vi "Await Queue Data Float.vi"(9 "Array":dbl[][](array[numeric]), 10 "Num Elements":i32, 11 "Spare Queue Float":refnum<queue>) -> (3 "Array Out":dbl[][](array[numeric]))   [LabVIEW 2018]
uses:
  Floating Pixel Data STYP.ctl
  Coordinate STYP.ctl
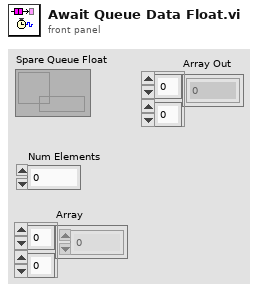
[diagram p1: front panel]
types:
  T1 = typedef "Floating Pixel Data STYP.ctl" = cluster{"Value":dbl, "Coordinate":T2}
  T2 = typedef "Coordinate STYP.ctl" = cluster{"X":i32, "Y":i32}
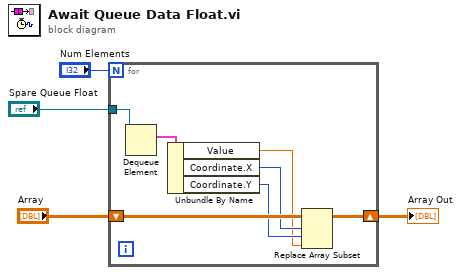
[diagram p0: block diagram]
diagram:
  n1 = for {
    N: "Num Elements" -> [_]
    tunnel: "Spare Queue Float" -> [w11]
    shift-right: [w5] -> w2
    shift-left: "Array" -> [w9]
    n2 = Dequeue Element(queue=w11) -> (element=w10:T1)  [unwired: 2 in, 3 out]
    n3 = Unbundle By Name(w10) -> ("Value"=w6:dbl, "Coordinate.X"=w8:i32, "Coordinate.Y"=w7:i32)
    n4 = Replace Array Subset(array=w9, new element=w6, index (row)=w8, index (col)=w7) -> (w5:dbl[][])
  }
  "Array Out" <- w2
